vi "OAT Shaft Centerline Plot.vi"(0 "picture":picture, 1 "picture\ndimensions (w,h)":cluster{"width":u32, "height":u32}, 2 "shaft centerline plot settings":T6={"cartesian grid cosmetics"={"line color"=7171459, "text color"=0, "tick length(3)"=3, "crossing axes"=FALSE, "visible grid?"=TRUE}, "XY plot cosmetics"={"plot color"=16711680, "XY plot type"=enum."connected points", "baseline"=0.0}, "desired font(Application)"=enum."Application Font", "[user-specified font]"={"Font Name:"="", "Size"=0, "Strikeout?"=FALSE, "Italic?"=FALSE, "Underline?"=FALSE, "Outline?"=FALSE, "Shadow?"=FALSE, "Bold?"=FALSE}} {"XY plot cosmetics"."baseline" format="%0.2f"}, 3 "cursor attributes":T7={"layout color"=852223, "active color"=16740820, "precision"=2, "BG transparent? (T)"=TRUE, "radius"=2}, 5 "DC gaps":cluster{"time/rev/rpm":dbl[], "DC gap":dbl[]}[](array[cluster]) {"DC gap" format="%.2f"; "time/rev/rpm" format="%.2f"}, 9 "clearance boundary settings":T3={"start point"=enum."bottom", " boundary"={"x axis"=0.0, "y axis"=0.0}}, 11 "error in (no error)":errorcluster, 12 "channel settings":T4={"shaft rotating direction"=0, "probe angles [deg]"={"X"=0, "Y"=90}} {"probe angles [deg]"."Y" max=360 step=1; "probe angles [deg]"."X" max=360 step=1; "shaft rotating direction" items=["CCW", "CW"]}, 13 "plot scale settings":T1, 14 "label settings":T2={"show label? (T)"=TRUE, "avoid overlap? (T)"=TRUE}) -> (4 "new picture":picture, 15 "error out":errorcluster)   [LabVIEW 2017]
doc: "LabVIEW no longer supports this VI. Use the SVX Shaft Centerline Plot VI instead. Draws a shaft centerline plot on a picture control. Shaft centerline plots display the averaged positions of the shaft center. Mount two transducers of the same type orthogonally, ninety degrees out of phase, to acquire data for a shaft centerline plot."
uses:
  <vilib>/addons/Sound and Vibration/Order Analysis/Backward Compatibility/SubVIs/OAT Polar Cursor Attributes.ctl
  <vilib>/picture/cartesn2.llb/XY Plot Type.ctl
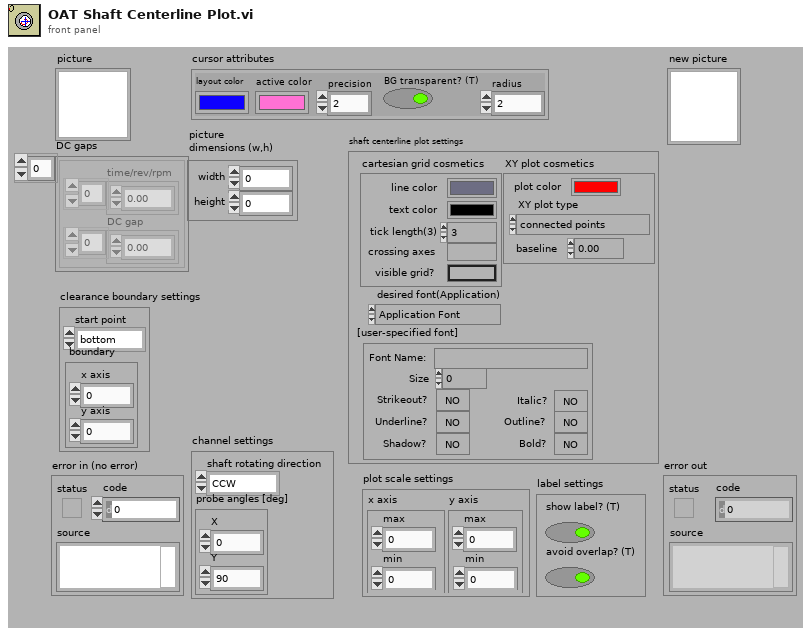
[diagram p1: front panel]
types:
  T1 = cluster{"x axis":cluster{"max":dbl, "min":dbl}, "y axis":cluster{"max":dbl, "min":dbl}}
  T2 = cluster{"show label? (T)":bool, "avoid overlap? (T)":bool}
  T3 = cluster{"start point":enum16{"top", "center", "bottom"}, " boundary":cluster{"x axis":dbl, "y axis":dbl}}
  T4 = cluster{"shaft rotating direction":u16, "probe angles [deg]":cluster{"X":u32, "Y":u32}}
  T5 = typedef "XY Plot Type.ctl" = enum16{"points", "squares", "circles", "connected points", "connected squares", "connected circles", "comb plot", "sized scatter plot", "sized-colored scatter plot", "min-max lines"}
  T6 = cluster{"cartesian grid cosmetics":cluster{"line color":u32, "text color":u32, "tick length(3)":i16, "crossing axes":bool, "visible grid?":bool}, "XY plot cosmetics":cluster{"plot color":u32, "XY plot type":T5, "baseline":dbl}, "desired font(Application)":enum16{"User-specified Font", "Application Font", "System Font", "Dialog Font"}, "[user-specified font]":cluster{"Font Name:":string, "Size":i16, "Strikeout?":bool, "Italic?":bool, "Underline?":bool, "Outline?":bool, "Shadow?":bool, "Bold?":bool}}
  T7 = typedef "OAT Polar Cursor Attributes.ctl" = cluster{"layout color":u32, "active color":u32, "precision":i16, "BG transparent? (T)":bool, "radius":i16}
  T8 = cluster{"x axis maxmin":cluster{"max":dbl, "min":dbl}, "y axis maxmin":cluster{"max":dbl, "min":dbl}}
  T9 = cluster{"Name":string, "Location":cluster{"mag":dbl, "phase":dbl}}[]
  T10 = cluster{"scale":cluster{"x axis maxmin":cluster{"max":dbl, "min":dbl}, "y axis maxmin":cluster{"max":dbl, "min":dbl}}, "x scale factors":cluster{"a":dbl, "b":dbl, "log?":bool}, "y scale factors":cluster{"a":dbl, "b":dbl, "log?":bool}}
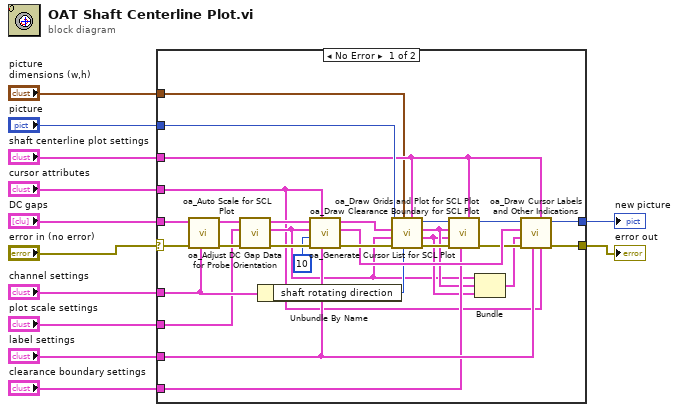
[diagram p0: block diagram]
diagram:
  n1 = case shown="No Error" "error in (no error)" {
    selector: "error in (no error)" -> [w25 w43]
    tunnel: [w24 w43] -> w11
    tunnel: "DC gaps" -> [w41 _]
    tunnel: "channel settings" -> [w27 _]
    tunnel: "label settings" -> [w28 _]
    tunnel: "cursor attributes" -> [w14 _]
    tunnel: "picture" -> [w35 w42]
    tunnel: "picture\ndimensions (w,h)" -> [w15 _]
    tunnel: "shaft centerline plot settings" -> [w26 _]
    tunnel: "clearance boundary settings" -> [w20 _]
    tunnel: [w23 w42] -> w2
    tunnel: "plot scale settings" -> [w21 _]
    frame No Error {
      n2 = call <vilib>:"oa_Adjust DC Gap Data for Probe Orientation.vi"("rotating settings"=w27, "error in (no error)"=w25, "DC Gap"=w41) -> ("error out"=w38:errorcluster, "DC Gap out"=w40:cluster{"X":dbl[], "Y":dbl[]}[])  [unwired: 7 in]
      n3 = call <vilib>:"oa_Auto Scale for SCL Plot.vi"("error in (no error)"=w38, "scale in"=w21, "DC Gap"=w40) -> ("error out"=w37:errorcluster, "scale"=w17:T8, "DC Gap out"=w39:cluster{"X":dbl[], "Y":dbl[]}[])  [unwired: 6 in]
      n4 = Unbundle By Name(w27) -> ("shaft rotating direction"=w22:u16)
      n5 = call <vilib>:"oa_Generate Cursor List for SCL Plot.vi"("label settings"=w28, "cursor attributes"=w14, "error in (no error)"=w37, "Max number of labels\nalong radius"=10 ("Max number of labels\nalong radius"), "scale"=w17, "DC Gap"=w39) -> ("error out"=w34:errorcluster, "Cursor List (EU position]"=w30:T9, "DC Gap out"=w36:cluster{"X":dbl[], "Y":dbl[]}[])  [unwired: 3 in]
      n6 = call <vilib>:"oa_Draw Grids and Plot for SCL Plot.vi"("shaft center line settings"=w26, "shaft rotating direction"=w22, "picture \ndimensions (w,h)"=w15, "error in (no error)"=w34, "scale"=w17, "DC Gap"=w36, "picture"=w35) -> ("error out"=w32:errorcluster, "y scale factors"=w18:cluster{"a":dbl, "b":dbl, "log?":bool}, "x scale factors"=w19:cluster{"a":dbl, "b":dbl, "log?":bool}, "new picture"=w33:picture)  [unwired: 1 in]
      n7 = call <vilib>:"oa_Draw Clearance Boundary for SCL Plot.vi"("shaft center line settings"=w26, "clearance boundary settings"=w20, "error in (no error)"=w32, "y scale factors"=w18, "x scale factors"=w19, "picture"=w33) -> ("error out"=w29:errorcluster, "new picture"=w31:picture)  [unwired: 4 in]
      n8 = Bundle("scale"=w17, "x scale factors"=w19, "y scale factors"=w18) -> (w16:T10)  [unwired: 1 in]
      n9 = call <vilib>:"oa_Draw Cursor Labels and Other Indications.vi"("cursor attributes"=w14, "shaft center line settings"=w26, "label settings"=w28, "error in (no error)"=w29, "scale info"=w16, "Cursor List (EU position]"=w30, "picture"=w31) -> ("error out"=w24:errorcluster, "new picture"=w23:picture)  [unwired: 3 in]
    }
    frame Error {
    }
  }
  "new picture" <- w2
  "error out" <- w11
